vi "Configure Frequency.vi"(8 "error in (no error)":errorcluster, 10 "Frequency":dbl, 11 "PM-EMP in":refnum<class "PM-EMP.lvclass">) -> (0 "error out":errorcluster, 3 "PM-EMP out":refnum<class "PM-EMP.lvclass">)   [LabVIEW 2020, in "PM-EMP.lvclass"]
doc: "Vi for configureting the frequency"
uses:
  PM-EMP.lvclass
  C:/Sandbox/Git_Sandbox/WiSpry Test Framework source code (LV20)/WiSpry Test Framework/Instruments/Instrument.lvclass
  C:/Sandbox/Git_Sandbox/WiSpry Test Framework source code (LV20)/WiSpry Test Framework/Instruments/Power Meter/Power Meter.lvclass
  Instrument.lvclass/Instrument.ctl
  Power Meter.lvclass/Power Meter.ctl
  Instrument.lvclass
  Power Meter.lvclass
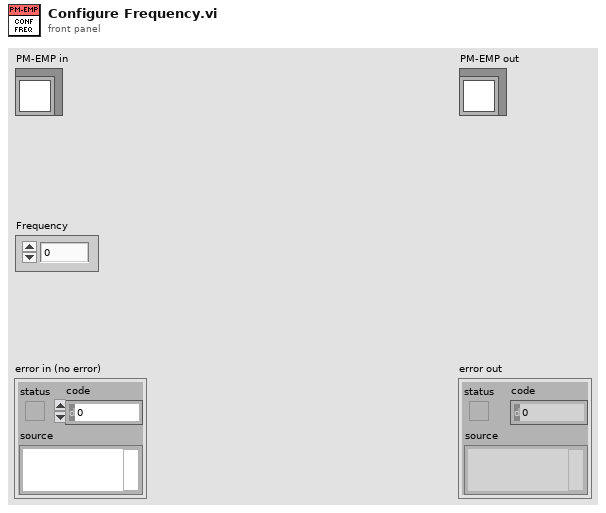
[diagram p1: front panel]
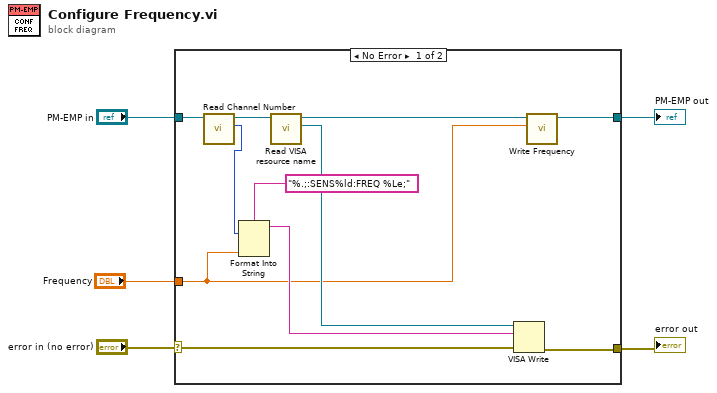
[diagram p0: block diagram]
diagram:
  n1 = case shown="No Error" "error in (no error)" {
    selector: "error in (no error)" -> [w14 w18]
    tunnel: [w16 w18] -> w4
    tunnel: "PM-EMP in" -> [w8 w17]
    tunnel: [w11 w17] -> w2
    tunnel: "Frequency" -> [w9 _]
    frame No Error {
      n2 = call-dynamic "Read Channel Number.vi"("Power Meter in"=w8) -> ("Channel Number"=w6:u8, "Power Meter out"=w7:refnum<class "PM-EMP.lvclass">)  [unwired: 9 in]
      n3 = Format Into String(format string="%.;:SENS%ld:FREQ %Le;", w6, w9) -> (resulting string=w12:string)  [unwired: 2 in, 1 out]
      n4 = call "Read VISA resource name.vi"("Instrument in"=w7) -> ("VISA resource name"=w15:refnum<visa-resource-name>, "Instrument out"=w10:refnum<class "PM-EMP.lvclass">)  [unwired: 9 in]
      n5 = VISA Write(VISA resource name=w15, write buffer=w12, error in (no error)=w14) -> (error out=w16:errorcluster)  [unwired: 2 out]
      n6 = call "Write Frequency.vi"("Frequency"=w9, "Power Meter in"=w10) -> ("Power Meter out"=w11:refnum<class "PM-EMP.lvclass">)  [unwired: 9 in]
    }
    frame Error {
    }
  }
  "error out" <- w4
  "PM-EMP out" <- w2
